vi "FTW-JSON-Interpret-String.vi"(1 "JSON String":string) -> (0 "LabVIEW String":string)   [LabVIEW 2015]
panel:
  # "Inputs"
  # "Outputs"
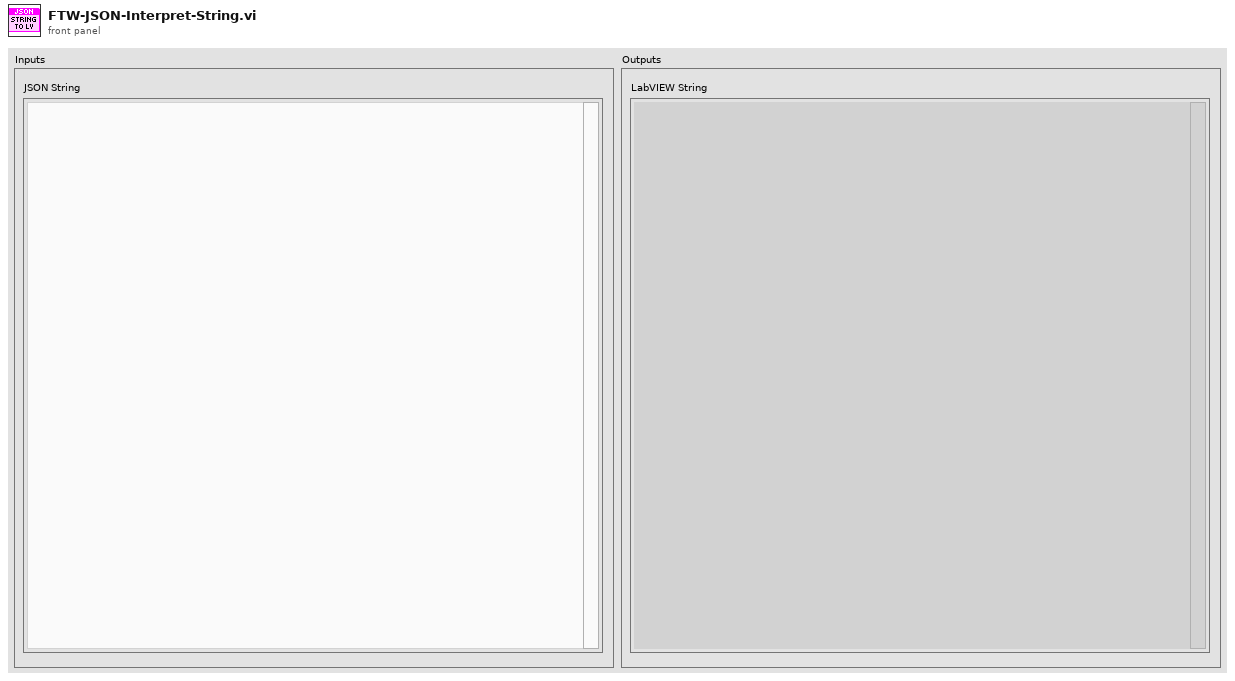
[diagram p1: front panel]
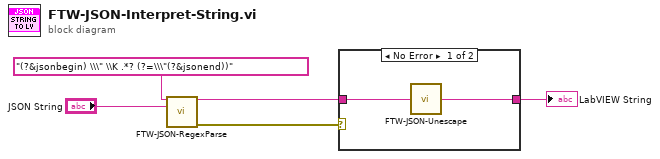
[diagram p0: block diagram]
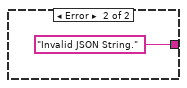
[diagram p2: hidden frame]
diagram:
  n1 = call "FTW-JSON-RegexParse.vi"("Regular Expression using JSON subroutines"="(?&jsonbegin) \\\" \\K .*? (?=\\\"(?&jsonend))" ("Regular Expression"), "Input String"="JSON String") -> ("Match"=w3:string, "error out"=w2:errorcluster)  [unwired: 9 in, 3 out]
  n2 = case shown="No Error" w2 {
    tunnel: [w7 "Invalid JSON String." ("Unescaped String")] -> w5
    tunnel: w3 -> [w6 _]
    frame No Error {
      n3 = call "FTW-JSON-Unescape.vi"("Escaped UTF-8 String"=w6) -> ("Unescaped String"=w7:string)
    }
    frame Error {
    }
  }
  "LabVIEW String" <- w5
